vi "SEDA Specific Entahalpy of Dry Air (J to Kg).vi"(1 "Tceg":dbl[unit]) -> (0 "SEDA":dbl[unit])   [LabVIEW 2018]
panel:
  out "Cp_DA or SHCDA":dbl[unit]
  out "Cp_DA or SHCDA":dbl[unit]
  out "SEDA\nSpecific Entahalpy of Dry Air\nSEDA=Cp_da*Tc;":dbl[unit](knob)
  out "Temprature Of Input Air\nKelvin Degree":dbl[unit](slide) scale=273.0..373.0
  out "Tk":dbl[unit]
  out "Temprature Of Input Air\nCentigrade Degree":dbl[unit](slide) scale=0.0..100.0
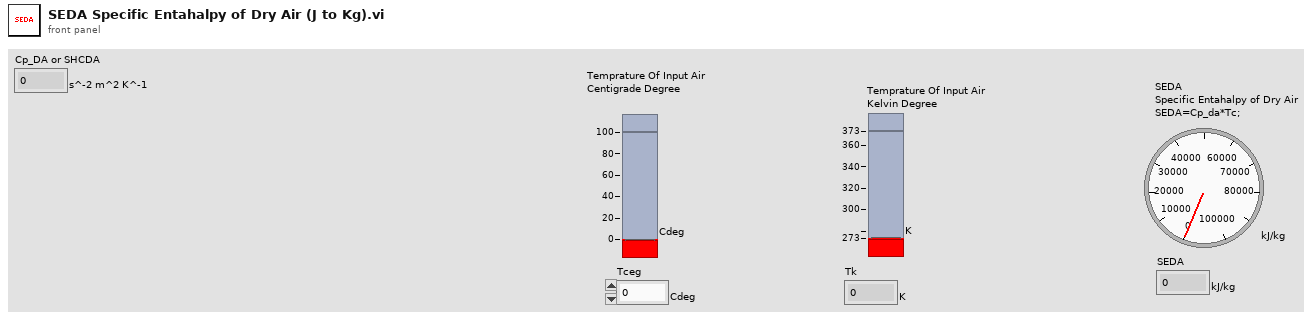
[diagram p1: front panel]
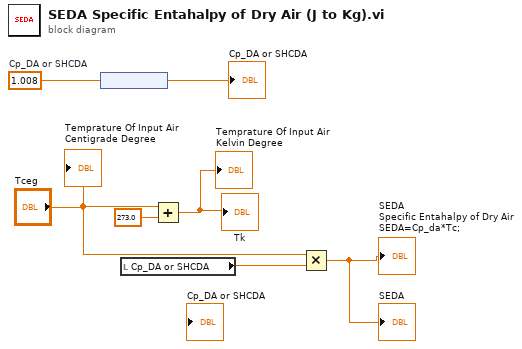
[diagram p0: block diagram]
diagram:
  w2 = 1.008  # Cp_DA or SHCDA
  n1 = node(w2) -> (→"Cp_DA or SHCDA":dbl[unit])
  n2 = local read "Cp_DA or SHCDA"() -> (w1:dbl[unit])
  n3 = Add(x="Tceg", y=dbl[unit] 273.0) -> (x+y=→"Tk" →"Temprature Of Input Air\nKelvin Degree":dbl[unit])
  n4 = Multiply(x="Tceg", y=w1) -> (x*y=→"SEDA\nSpecific Entahalpy of Dry Air\nSEDA=Cp_da*Tc;" →"SEDA":dbl[unit])
  "Temprature Of Input Air\nCentigrade Degree" <- "Tceg"
